vi "3D transpose (SubVI).vi"(7 "Enum":T1(ring), 11 "3D in":u16[][][](array[numeric])) -> (3 "3D out":u16[][][](array[numeric]))   [LabVIEW 2024]
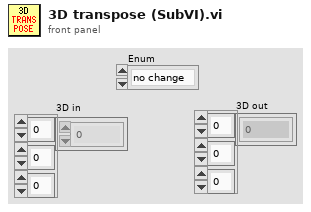
[diagram p1: front panel]
types:
  T1 = enum16{"no change", "zyx->zxy", "zyx->xyz", "zyx->yzx", "zyx->yxz", "zyx->xzy"}
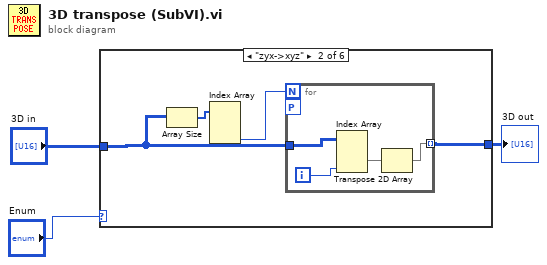
[diagram p0: block diagram]
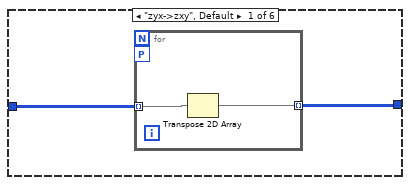
[diagram p2: hidden frame]
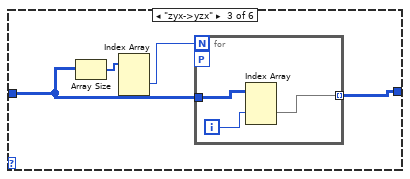
[diagram p3: hidden frame]
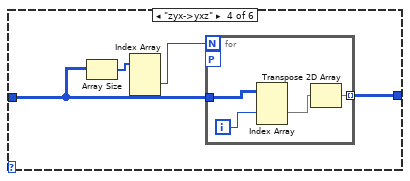
[diagram p4: hidden frame]
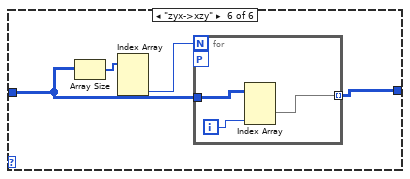
[diagram p6: hidden frame]
diagram:
  n1 = case shown="\"zyx->xyz\"" "Enum" {
    tunnel: "3D in" -> [w5 w10 w18 w25 w31 w33]
    tunnel: [w4 w9 w17 w24 w31 w32] -> w1
    frame "zyx->zxy", Default {
      n2 = for {
        tunnel: w5 -> [w7] mode=indexing
        tunnel: [w6] -> w4 mode=indexing
        workers-P: _ -> [_]
        n3 = Transpose 2D Array(2D array=w7) -> (transposed array=w6:u16[][])
      }
    }
    frame "zyx->xyz" {
      n4 = Array Size(array=w10) -> (size(s)=w11:i32[])
      n5 = Index Array(array=w11) -> (element #3=w8:i32)  [unwired: 3 in, 2 out]
      n6 = for {
        N: w8 -> [_]
        tunnel: w10 -> [w15]
        tunnel: [w12] -> w9 mode=indexing
        workers-P: _ -> [_]
        i -> [w13]
        n7 = Index Array(array=w15, index (dim 2)=w13) -> (element=w14:u16[][])  [unwired: 2 in]
        n8 = Transpose 2D Array(2D array=w14) -> (transposed array=w12:u16[][])
      }
    }
    frame "zyx->yzx" {
      n9 = Array Size(array=w18) -> (size(s)=w19:i32[])
      n10 = Index Array(array=w19) -> (element #2=w16:i32)  [unwired: 3 in, 2 out]
      n11 = for {
        N: w16 -> [_]
        tunnel: w18 -> [w22]
        tunnel: [w21] -> w17 mode=indexing
        workers-P: _ -> [_]
        i -> [w20]
        n12 = Index Array(array=w22, index (dim 1)=w20) -> (element=w21:u16[][])  [unwired: 2 in]
      }
    }
    frame "zyx->yxz" {
      n13 = Array Size(array=w25) -> (size(s)=w26:i32[])
      n14 = Index Array(array=w26) -> (element #2=w23:i32)  [unwired: 3 in, 2 out]
      n15 = for {
        N: w23 -> [_]
        tunnel: w25 -> [w30]
        tunnel: [w28] -> w24 mode=indexing
        workers-P: _ -> [_]
        i -> [w27]
        n16 = Index Array(array=w30, index (dim 1)=w27) -> (element=w29:u16[][])  [unwired: 2 in]
        n17 = Transpose 2D Array(2D array=w29) -> (transposed array=w28:u16[][])
      }
    }
    frame "no change" {
    }
    frame "zyx->xzy" {
      n18 = Array Size(array=w33) -> (size(s)=w35:i32[])
      n19 = Index Array(array=w35) -> (element #3=w34:i32)  [unwired: 3 in, 2 out]
      n20 = for {
        N: w34 -> [_]
        tunnel: w33 -> [w38]
        tunnel: [w37] -> w32 mode=indexing
        workers-P: _ -> [_]
        i -> [w36]
        n21 = Index Array(array=w38, index (dim 2)=w36) -> (element=w37:u16[][])  [unwired: 2 in]
      }
    }
  }
  "3D out" <- w1
